vi "Configure.vi"(8 "error in":errorcluster, 10 "name":string, 11 "nPAS in":refnum<class "nPAS.lvclass">) -> (0 "error out":errorcluster, 3 "nPAS out":refnum<class "nPAS.lvclass">)   [LabVIEW 2017, in "gPAS Library.lvlib" / "nPAS.lvclass"]
doc: "Configure the instrument class. If there is no config file specified, an error"
uses:
  nPAS.lvclass
  C:/Program Files (x86)/National Instruments/LabVIEW 2017/vi.lib/MSR Consulting, LLC/General Reuse/PAS/Main/PAS.lvclass
  C:/Program Files (x86)/National Instruments/LabVIEW 2017/vi.lib/MSR Consulting, LLC/General Reuse/Instrument/Instrument.lvclass
  Session/Raw FPGA/FPGA Session.lvclass
  C:/Program Files (x86)/National Instruments/LabVIEW 2017/vi.lib/MSR Consulting, LLC/General Reuse/Session APIs/_Session Fwk/Session - Root.lvclass
  Commands/Update Speaker Vscale Cmd/Update Speaker Vscale CMD.lvclass
  C:/Program Files (x86)/National Instruments/LabVIEW 2017/vi.lib/MSR Consulting, LLC/General Reuse/Command/Command.lvclass
  Commands/Update Chirp Cmd/Update Chirp CMD.lvclass
  Commands/Change Laser Frequency Cmd/Change Laser Frequency CMD.lvclass
  Commands/Change Speaker State Cmd/Change Speaker State CMD.lvclass
  C:/Program Files (x86)/National Instruments/LabVIEW 2017/vi.lib/MSR Consulting, LLC/General Reuse/PAS/Commands/Change Speaker State CMD/Change Speaker State CMD.lvclass
  Commands/Change Laser Frequency Cmd/Change Laser Frequency CMD.lvclass/Change Laser Frequency CMD.ctl
  <vilib>/MSR Consulting, LLC/General Reuse/PAS/Commands/Change Speaker State CMD/Change Speaker State CMD.lvclass/Change Speaker State CMD.ctl
  Session/Raw FPGA/FPGA Session.lvclass/FPGA Session.ctl
  <vilib>/MSR Consulting, LLC/General Reuse/Instrument/Instrument.lvclass/Instrument.ctl
  <vilib>/MSR Consulting, LLC/General Reuse/PAS/Main/PAS.lvclass/PAS.ctl
  nPAS.lvclass/nPAS.ctl
  Commands/Update Chirp Cmd/Update Chirp CMD.lvclass/Update Chirp CMD.ctl
  <vilib>/MSR Consulting, LLC/General Reuse/Session APIs/File Access/Config Data/Config Data.lvclass/Config Data.ctl
  Commands/Update Speaker Vscale Cmd/Update Speaker Vscale CMD.lvclass/Update Speaker Vscale CMD.ctl
  <vilib>/MSR Consulting, LLC/General Reuse/PAS/Commands/Change Speaker State CMD/Write state.vi
  Commands/Change Laser Frequency Cmd/Write Cell.vi
  Commands/Change Laser Frequency Cmd/Write f.vi
  Session/Raw FPGA/Read FPGA Ref.vi
  <vilib>/MSR Consulting, LLC/General Reuse/Instrument/Read Cfg Session.vi
  <vilib>/MSR Consulting, LLC/General Reuse/PAS/Main/Read Chirp.vi
  <vilib>/MSR Consulting, LLC/General Reuse/Instrument/Read CMD.vi
  Commands/Update Chirp Cmd/Write fcenter.vi
  Commands/Update Chirp Cmd/Write df.vi
  <vilib>/MSR Consulting, LLC/General Reuse/Session APIs/File Access/Config Data/Accessors/Read Ref.vi
  Commands/Update Speaker Vscale Cmd/Write Voffset.vi
  Commands/Update Speaker Vscale Cmd/Write Vscale.vi
  <vilib>/MSR Consulting, LLC/General Reuse/Instrument/Read Log Session.vi
  <vilib>/MSR Consulting, LLC/General Reuse/PAS/Main/Write Speaker State CMD.vi
  <vilib>/MSR Consulting, LLC/General Reuse/PAS/Main/Get Speaker State.vi
  <vilib>/Utility/config.llb/Read Key (Double).vi
  <vilib>/Utility/error.llb/Error Cluster From Error Code.vi
  <vilib>/rvi/errors/niLvFpgaAdjustHostInterfaceError.vi
  <vilib>/MSR Consulting, LLC/General Reuse/PAS/Main/PAS.lvclass
  FPGA Ref.ctl
  <vilib>/MSR Consulting, LLC/General Reuse/Session APIs/File Access/Config Data/Config Data.lvclass
  <vilib>/MSR Consulting, LLC/General Reuse/Command/Command.lvclass
  <vilib>/MSR Consulting, LLC/General Reuse/Session APIs/_Session Fwk/Session - Root.lvclass
  <vilib>/rvi/interface/nirviReadWriteControl/nirviReadWriteControl.xnode
  FPGA Bitfiles/server_v1_2_1_4.lvbitx
  <vilib>/rvi/interface/nirviMethod/nirviMethod.xnode
  <vilib>/MSR Consulting, LLC/General Reuse/Session APIs/Session Log/System Log.lvclass
  <vilib>/Utility/config.llb/NI_LVConfig.lvlib
  NiFpgaLv.dll
  <vilib>/FPGAPlugInAG/cRIO-9081/niLvFpga_WriteFifo_cRIO-9081.vi
  <vilib>/rvi/errors/niLvFpgaMergeErrorWithErrorCode.vi
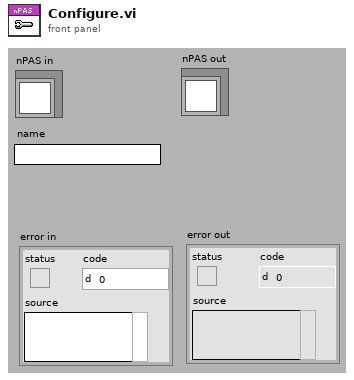
[diagram p1: front panel]
types:
  T1 = typedef "Session - Root.lvclass/Session Handle.ctl" = refnum<data-value>
  T2 = typedef "FPGA Ref.ctl" = refnum<k20>
  T3 = typedef "NI_LVConfig.lvlib/Config Data RefNum.ctl" = refnum<k1>
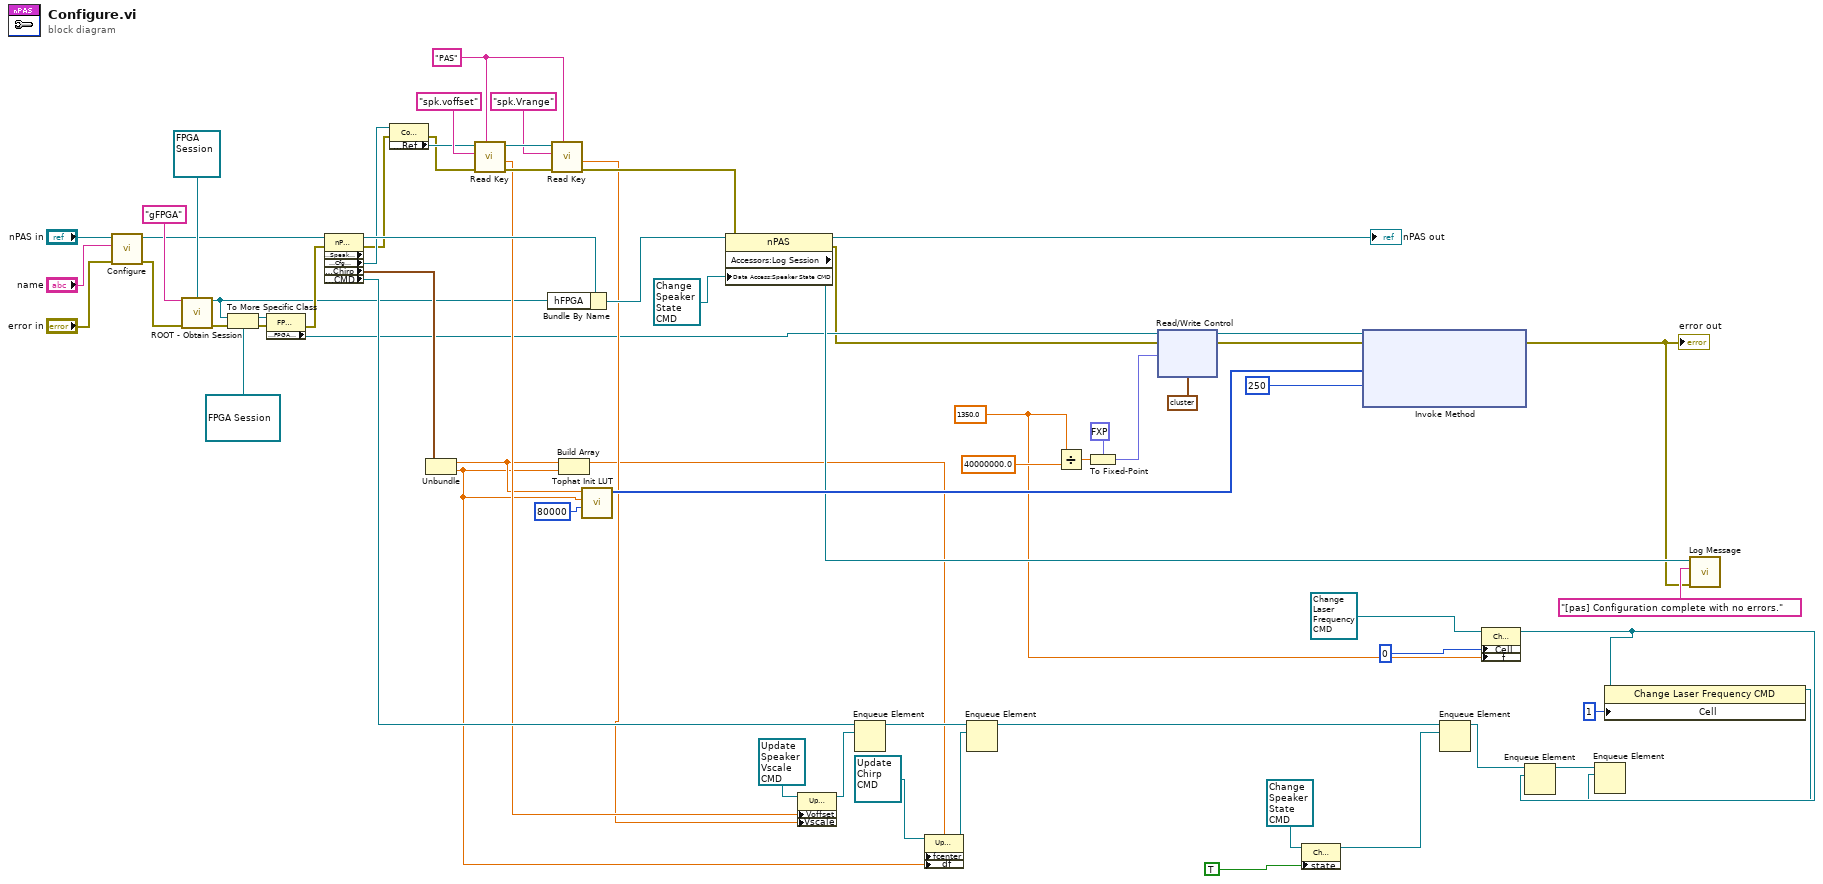
[diagram p0: block diagram]
diagram:
  w40 = "PAS" ("section")
  w12 = 1350.0 ("x")
  n1 = call-parent "Configure.vi"("error in"="error in", "name"="name", "PAS in"="nPAS in") -> ("error out"=w51:errorcluster, "PAS out"=w45:refnum<class "nPAS.lvclass">)  [unwired: 7 in]
  n2 = call <vilib>:"ROOT - Obtain Session.vi"("Session Name ()"="gFPGA", "OBJ - Session"=refnum<class "FPGA Session.lvclass"> refnum ("FPGA Session.lvclass"), "error in (no error)"=w51) -> ("Session Handle"=w15:T1, "error out"=w58:errorcluster)  [unwired: 10 in, 1 out]
  n3 = To More Specific Class(target class=refnum<data-value> refnum ("hFPGA"), reference=w15, error in=w58) -> (specific class reference=w61:refnum<data-value>, error out=w57:errorcluster)
  n4 = property class="FPGA Session"(reference=w61, error in=w57) -> (error out=w38:errorcluster, "Accessors:FPGA Ref"=w5:T2)  [unwired: 1 out]
  n5 = property class="nPAS" props=["Data Access:Speaker State", "Accessors:Cfg Session", "Data Access:Chirp", "Accessors:CMD"](reference=w45, error in=w38) -> (reference out=w44:refnum<class "nPAS.lvclass">, error out=w33:errorcluster, "Accessors:Cfg Session"=w35:refnum<data-value>, "Data Access:Chirp"=w37:cluster{"f_center":dbl, "bandwidth":dbl}, "Accessors:CMD"=w29:refnum<queue>)  [unwired: 1 out]
  n6 = property class="Config Data"(reference=w35, error in=w33) -> (error out=w32:errorcluster, "Accessors:Ref"=w34:T3)  [unwired: 1 out]
  n7 = Unbundle(w37) -> ("f_center"=w22:dbl, "bandwidth"=w21:dbl)
  n8 = call-poly <vilib>:"Read Key.vi"("section"=w40, "error in (no error)"=w32, "key"="spk.voffset" ("section"), "refnum"=w34) -> ("error out"=w36:errorcluster, "value"=w27:dbl, "refnum out"=w43:T3)  [unwired: 4 in, 1 out]
  n9 = Bundle By Name(cluster=w44, "hFPGA"=w15) -> (w49:refnum<class "nPAS.lvclass">)
  n10 = call-poly <vilib>:"Read Key.vi"("section"=w40, "error in (no error)"=w36, "key"="spk.Vrange", "refnum"=w43) -> ("error out"=w31:errorcluster, "value"=w26:dbl)  [unwired: 4 in, 2 out]
  n11 = Build Array(w22, w21) -> ()  [unwired: 1 out]
  n12 = call <vilib>:"Tophat Init LUT.vi"("Number of  Elements"=80000, "Df"=w21, "f0"=w22) -> ("Init Data Out"=w52:i16[])  [unwired: 6 in]
  n13 = property class="nPAS"(reference=w49, error in=w31, "Data Access:Speaker State CMD"=refnum<class "Change Speaker State CMD.lvclass"> refnum ("gPAS Library.lvlib:Change Speaker State CMD")) -> (reference out=→"nPAS out":refnum<class "nPAS.lvclass">, error out=w4:errorcluster, "Accessors:Log Session"=w47:T1)
  n14 = property class="Update Speaker Vscale CMD"(reference=refnum<class "Update Speaker Vscale CMD.lvclass"> refnum ("gPAS Library.lvlib:Update Speaker Vscale CMD"), "Voffset"=w27, "Vscale"=w26) -> (reference out=w25:refnum<class "Update Speaker Vscale CMD.lvclass">)  [unwired: 1 in, 1 out]
  n15 = Enqueue Element(queue=w29, element=w25) -> (queue out=w24:refnum<queue>)  [unwired: 2 in, 2 out]
  n16 = property class="Update Chirp CMD"(reference=refnum<class "Update Chirp CMD.lvclass"> refnum ("gPAS Library.lvlib:Update Chirp CMD"), "fcenter"=w22, "df"=w21) -> (reference out=w20:refnum<class "Update Chirp CMD.lvclass">)  [unwired: 1 in, 1 out]
  n17 = Enqueue Element(queue=w24, element=w20) -> (queue out=w17:refnum<queue>)  [unwired: 2 in, 2 out]
  n18 = Divide(x=w12, y=40000000.0) -> (x/y=w55:dbl)
  n19 = To Fixed-Point(fixed-point type=fxp<+,32,0> 0.0 ("f0"), number=w55) -> (fixed-point=w30:fxp<+,32,0>)
  n20 = xnode "Read/Write Control"("FPGA VI Reference In"=w5, "error in"=w4, "f0"=w30, "Speaker"=cluster{"Vscale":fxp<+,32,0>, "Offset":i16} {"Vscale"=0.10000000009313226, "Offset"=0}) -> ("FPGA VI Reference Out"=w3:T2, "error out"=w2:errorcluster)
  n21 = property class="Change Speaker State CMD"(reference=refnum<class "Change Speaker State CMD.lvclass"> refnum ("gPAS Library.lvlib:Change Speaker State CMD"), "state"=TRUE ("State")) -> (reference out=w16:refnum<class "Change Speaker State CMD.lvclass">)  [unwired: 1 in, 1 out]
  n22 = xnode "Invoke Method"("FPGA VI Reference In"=w3, "error in"=w2, "Data"=w52, "Timeout (ms)"=250) -> ("error out"=w1:errorcluster)  [unwired: 2 out]
  "error out" <- w1
  n23 = Enqueue Element(queue=w17, element=w16) -> (queue out=w11:refnum<queue>)  [unwired: 2 in, 2 out]
  n24 = property class="Change Laser Frequency CMD"(reference=refnum<class "Change Laser Frequency CMD.lvclass"> refnum ("gPAS Library.lvlib:Change Laser Frequency CMD"), "Cell"=u8 0, "f"=w12) -> (reference out=w9:refnum<class "Change Laser Frequency CMD.lvclass">)  [unwired: 1 in, 1 out]
  n25 = Enqueue Element(queue=w11, element=w9) -> (queue out=w10:refnum<queue>)  [unwired: 2 in, 2 out]
  n26 = property class="Change Laser Frequency CMD"(reference=w9, "Cell"=u8 1) -> (reference out=w7:refnum<class "Change Laser Frequency CMD.lvclass">)  [unwired: 1 in, 1 out]
  n27 = Enqueue Element(queue=w10, element=w7) -> ()  [unwired: 2 in, 3 out]
  n28 = call <vilib>:"Log Message.vi"("error in"=w1, "MSG In"="[pas] Configuration complete with no errors.", "session in"=w47) -> ()  [unwired: 7 in, 2 out]
